vi "TDMStoAVI.vi"(0 "TDMS Path":path, 1 "Codec":string, 5 "AVI Out Path":path, 7 "Frames Per Second":u32, 11 "error in (no error)":errorcluster, 12 "Quality":i32, 13 "Image Type":u16) -> (15 "error out":errorcluster)   [LabVIEW 2023]
uses:
  Program Files/NI/LVAddons/niimaqdx/1/examples/Vision Acquisition/NI-IMAQdx/Stream to Disk/SubVIs/TDMS File Initialization (Read).vi
panel:
  in  "OK Button":bool
  in  "Stop Conversion":bool
  out "Percent Done":dbl
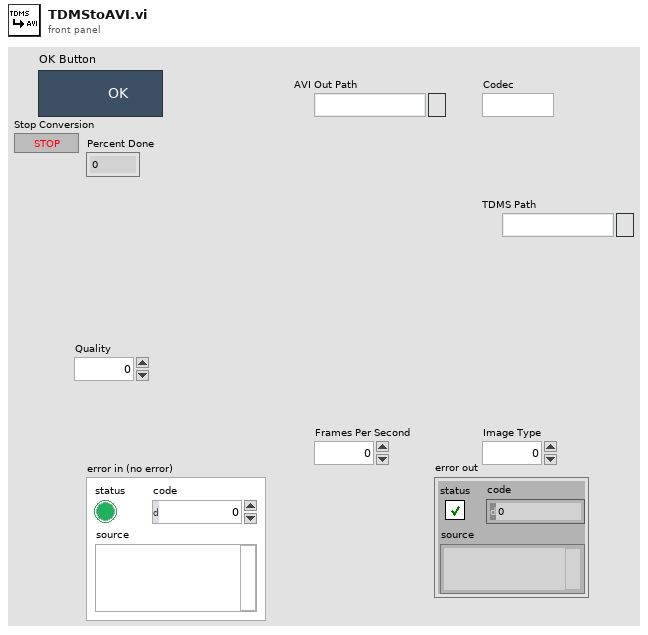
[diagram p1: front panel]
types:
  T1 = typedef "IMAQ Image.ctl" = refnum<image>
  T2 = typedef "TDMS Read Data.ctl" = cluster{"Image Type":T3, "Width":u32, "Height":u32, "Pixels per Image":u32, "Total Width":u32, "Left Offset":u32, "Image":T1}
  T3 = typedef "Image Type" = u32
  T4 = typedef "IMAQ AVI2 Refnum.ctl" = refnum<k20>
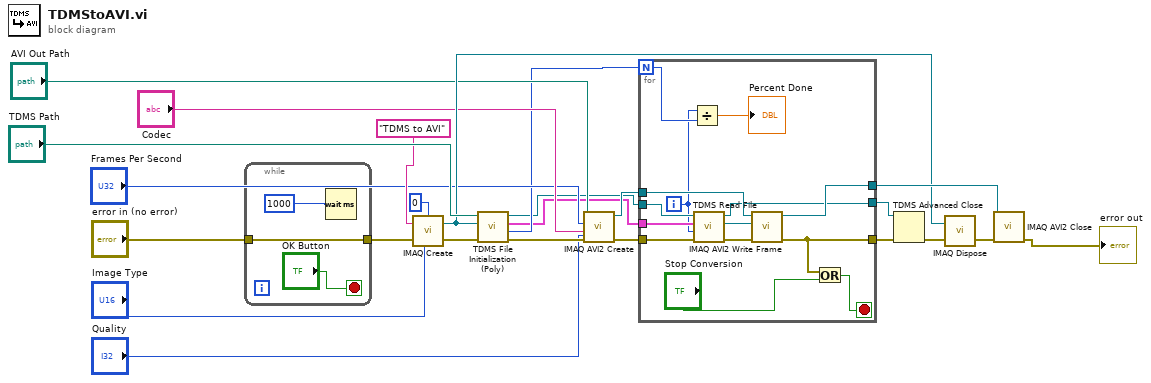
[diagram p0: block diagram]
diagram:
  n1 = while {
    tunnel: "error in (no error)" -> [w27]
    tunnel: [w27] -> w1
    stop <- "OK Button" stop-if-true
    n2 = Wait (ms)(milliseconds to wait=u32 1000) -> ()  [unwired: 1 out]
  }
  n3 = call "IMAQ Create"("Border Size"=0, "Image Name"="TDMS to AVI", "Image Type"="Image Type", "error in (no error)"=w1) -> ("New Image"=w20:T1, "error out"=w14:errorcluster)  [unwired: 1 out]
  n4 = call-poly "TDMS File Initialization (Poly).vi"("error in (no error)"=w14, "Image In"=w20, "File Path"="TDMS Path") -> ("error out"=w24:errorcluster, "Number of Images in TDMS File"=w6:u32, "Read Settings"=w5:T2, "TDMS Refnum Out"=w4:refnum<k34>)  [unwired: 5 in]
  n5 = call "IMAQ AVI2 Create"("Quality"="Quality", "error in (no error)"=w24, "Codec"="Codec", "Frames Per Second"="Frames Per Second", "AVI Path"="AVI Out Path") -> ("error out"=w10:errorcluster, "AVI Refnum"=w9:T4)  [unwired: 5 in]
  n6 = for {
    N: w6 -> [w35]
    tunnel: w10 -> [w41]
    tunnel: w4 -> [w40]
    tunnel: w5 -> [w39]
    tunnel: w9 -> [w38]
    tunnel: [w30] -> w16
    tunnel: [w36] -> w21
    tunnel: [w33] -> w17
    i -> [w31]
    stop <- w28 stop-if-true
    n7 = Divide(x=w31, y=w35) -> (x/y=→"Percent Done":dbl)
    n8 = call "TDMS Read File.vi"("error in"=w41, "Image Index"=w31, "Read Settings"=w39, "TDMS Refnum In"=w40) -> ("error out"=w37:errorcluster, "Image"=w32:T1, "TDMS Refnum Out"=w33:refnum<k34>)  [unwired: 4 in, 1 out]
    n9 = call "IMAQ AVI2 Write Frame"("error in (no error)"=w37, "Image"=w32, "AVI Refnum"=w38) -> ("error out"=w30:errorcluster, "AVI Refnum (duplicate)"=w36:T4)  [unwired: 6 in, 1 out]
    n10 = Or(x=w30, y="Stop Conversion") -> (x .or. y?=w28:bool)
  }
  n11 = TDMS Advanced Close(8:w16, 11:w17) -> (0:w18:errorcluster)  [unwired: 2 in, 1 out]
  n12 = call "IMAQ Dispose"("Image"=w20, "error in (no error)"=w18) -> ("error out"=w19:errorcluster)  [unwired: 4 in]
  n13 = call "IMAQ AVI2 Close"("error in (no error)"=w19, "AVI Refnum"=w21) -> ("error out"=→"error out":errorcluster)  [unwired: 9 in]
